vi "FixCodeSpacing.vi"(11 "Code":string) -> (3 "Cleaned":string)   [LabVIEW 2020]
panel:
  out "Array 2":i32[](array[numeric])
  out "Array":i32[](array[numeric])
  out "Indents":i32[](array[numeric])
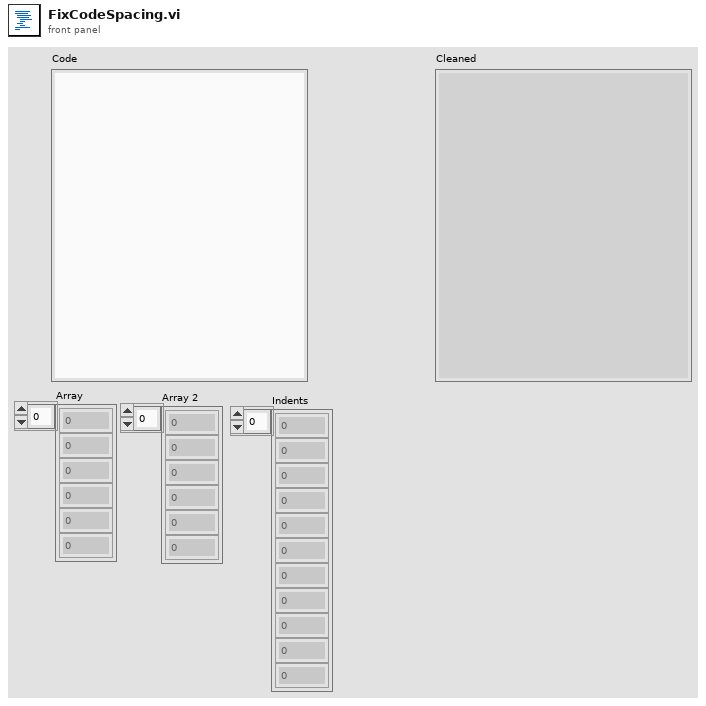
[diagram p1: front panel]
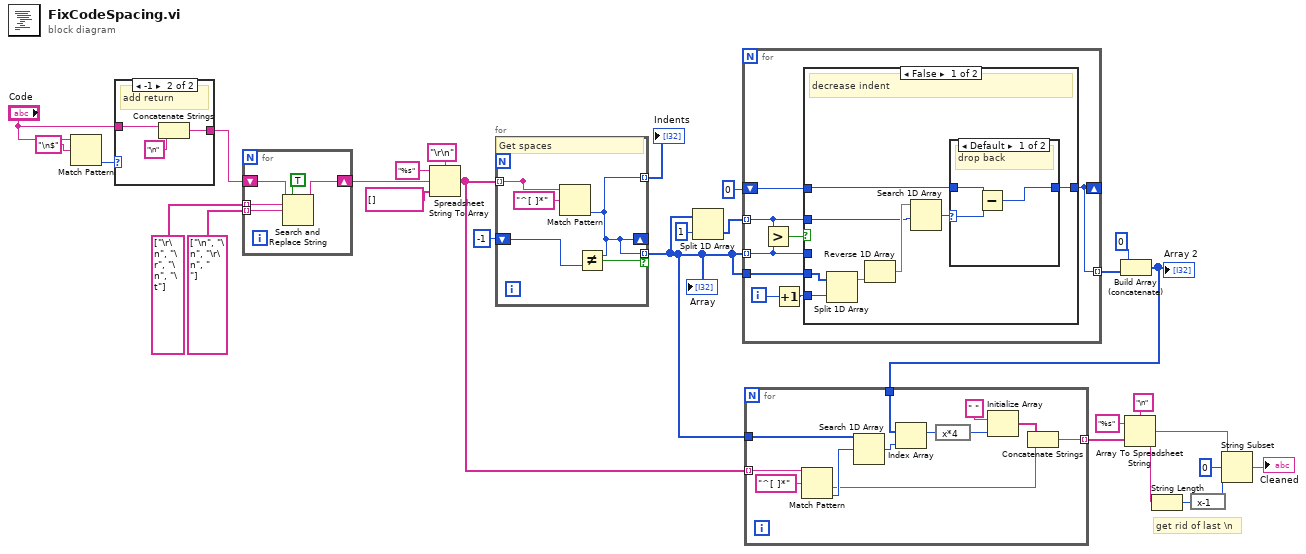
[diagram p0: block diagram]
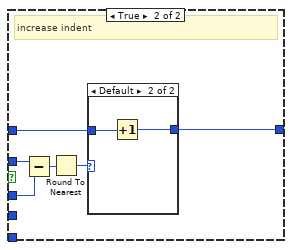
[diagram p4: hidden frame]
diagram:
  # "get rid of last \\n"
  n1 = Match Pattern(string="Code", regular expression="\n$" ("search string")) -> (offset past match=w3:i32)  [unwired: 1 in, 3 out]
  n2 = case shown="-1" w3 {
    tunnel: "Code" -> [w29 w32]
    tunnel: [w29 w30] -> w1
    frame Default {
    }
    frame -1 {
      # "add return"
      n3 = Concatenate Strings(w32, "\n" ("search string")) -> (w30:string)
    }
  }
  n4 = for {
    tunnel: string[] ["\r\n", "\r", "\n", "\t"] -> [w35] mode=indexing
    tunnel: string[] ["\n", "\n", "\r\n", "    "] -> [w34] mode=indexing
    shift-right: [w33] -> w22
    shift-left: w1 -> [w37]
    n5 = Search and Replace String(replace all?=TRUE ("replace all? (F)"), input string=w37, search string=w35, replace string=w34) -> (result string=w33:string)  [unwired: 4 in, 3 out]
  }
  n6 = Spreadsheet String To Array(delimiter (Tab)="\r\n" ("replace string (\"\")"), format string="%s", spreadsheet string=w22, array type (2D Dbl)=string[] []) -> (array=w16:string[])
  n7 = for {
    tunnel: [w42] -> _ mode=indexing
    tunnel: w16 -> [w42] mode=indexing
    tunnel: [w39] -> w23 mode=indexing
    shift-right: [w39] -> _
    shift-left: -1 ("offset past match") -> [w40]
    tunnel: [w39] -> w17 mode=indexing if=w38
    # "Get spaces"
    n8 = Match Pattern(string=w42, regular expression="^[ ]*") -> (offset past match=w39:i32)  [unwired: 1 in, 3 out]
    n9 = Not Equal?(x=w39, y=w40) -> (x != y?=w38:bool)
  }
  "Indents" <- w23
  "Array" <- w17
  n10 = Split 1D Array(array=w17, index=1) -> (second subarray=w19:i32[])  [unwired: 1 out]
  n11 = for {
    tunnel: w17 -> [w44] mode=indexing
    tunnel: w19 -> [w48] mode=indexing
    shift-right: [w43] -> _
    shift-left: 0 ("n") -> [w49]
    tunnel: w17 -> [w47]
    tunnel: [w43] -> w12 mode=indexing
    i -> [w46]
    n12 = Greater?(x=w48, y=w44) -> (0:w50:bool)
    n13 = Increment(x=w46) -> (x+1=w45:i32)
    n14 = case shown="False" w50 {
      tunnel: w49 -> [w57 w67]
      tunnel: [w56 w68] -> w43
      tunnel: w48 -> [w54 w64]
      tunnel: w47 -> [w53 _]
      tunnel: w45 -> [w51 _]
      tunnel: w44 -> [_ w63]
      frame False {
        # "decrease indent"
        n15 = Split 1D Array(array=w53, index=w51) -> (first subarray=w52:i32[])  [unwired: 1 out]
        n16 = Reverse 1D Array(array=w52) -> (reversed array=w55:i32[])
        n17 = Search 1D Array(1D array=w55, element=w54) -> (index of element=w58:i32)  [unwired: 1 in]
        n18 = case shown="Default" w58 {
          selector: w58 -> [w60 _]
          tunnel: w57 -> [w61 w62]
          tunnel: [w59 w62] -> w56
          frame Default {
            # "drop back"
            n19 = Subtract(x=w61, y=w60) -> (x-y=w59:i32)
          }
          frame -1 {
            # "not aligned"
          }
        }
      }
      frame True {
        # "increase indent"
        n20 = Subtract(x=w64, y=w63) -> (x-y=w65:i32)
        n21 = Round To Nearest(number=w65) -> (nearest integer value=w66:i32)
        n22 = case shown="Default" w66 {
          tunnel: w67 -> [w69 w71]
          tunnel: [w69 w70] -> w68
          frame 0, 1 {
          }
          frame Default {
            n23 = Increment(x=w71) -> (x+1=w70:i32)
          }
        }
      }
    }
  }
  n24 = Build Array (concatenate)(0 ("n"), w12) -> (w10:i32[])
  "Array 2" <- w10
  n25 = for {
    tunnel: w17 -> [w81]
    tunnel: w16 -> [w82] mode=indexing
    tunnel: [w75] -> w15 mode=indexing
    tunnel: w10 -> [w73]
    n26 = Match Pattern(string=w82, regular expression="^[ ]*") -> (after substring=w76:string, offset past match=w80:i32)  [unwired: 1 in, 2 out]
    n27 = Search 1D Array(1D array=w81, element=w80) -> (index of element=w79:i32)  [unwired: 1 in]
    n28 = Index Array(array=w73, index=w79) -> (element=w72:i32)
    n29 = expression code="x*4"(w72) -> (w74:i32)
    n30 = Initialize Array(" " ("regular expression"), w74) -> (w77:string[])
    n31 = Concatenate Strings(w77, w76) -> (w75:string)
  }
  n32 = Array To Spreadsheet String(delimiter (Tab)="\n" ("replace string (\"\")"), array=w15, 3:"%s" ("format string")) -> (spreadsheet string=w7:string)
  n33 = String Length(string=w7) -> (length=w6:i32)
  n34 = expression code="x-1"(w6) -> (w5:i32)
  n35 = String Subset(string=w7, offset (0)=0, length (rest)=w5) -> (substring=→"Cleaned":string)
